vi "Save_Header.vi"() -> ()   [LabVIEW 2018]
uses:
  RxTx/CCS_RxTx.lvclass
  Save Image/Save Image.lvclass
  Channel/Channel.lvclass
panel:
  in  "Stop Button":bool
  out "error out":errorcluster
  in  "Save Image out":refnum<class "Save Image.lvclass">
  in  "RxTx.lvclass":refnum<class "CCS_RxTx.lvclass">
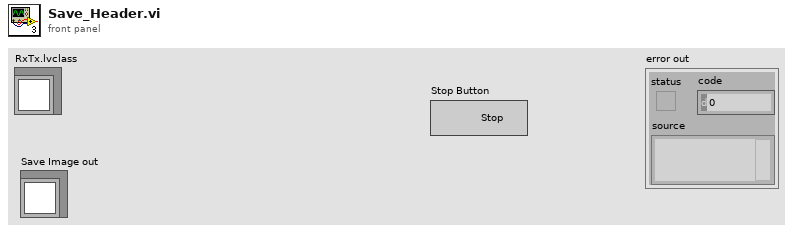
[diagram p1: front panel]
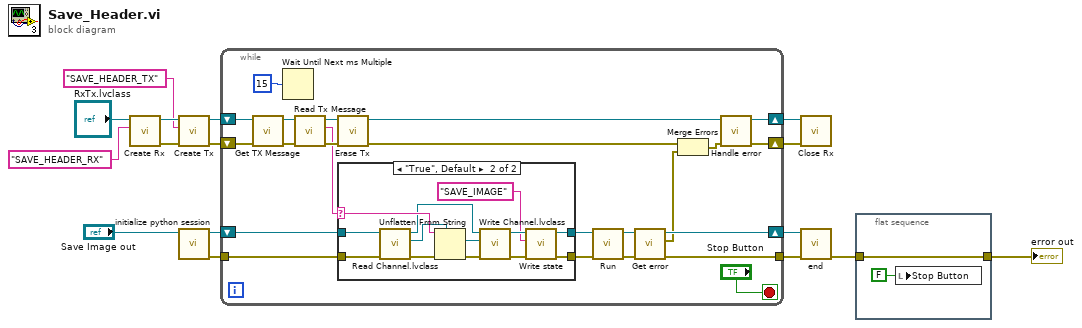
[diagram p0: block diagram]
diagram:
  n1 = call "Create Rx.vi"("Reader Name"="SAVE_HEADER_RX", "RxTx in"="RxTx.lvclass") -> ("error out"=w10:errorcluster, "RxTx out"=w11:refnum<class "CCS_RxTx.lvclass">)  [unwired: 8 in]
  n2 = call "Create Tx.vi"("error in (no error)"=w10, "Writer Name"="SAVE_HEADER_TX" ("Reader Name"), "RxTx in"=w11) -> ("error out"=w3:errorcluster, "RxTx out"=w4:refnum<class "CCS_RxTx.lvclass">)  [unwired: 7 in]
  n3 = call "initialize python session.vi"("Save Image in"="Save Image out") -> ("error out"=w7:errorcluster, "Save Image out"=w14:refnum<class "Save Image.lvclass">)  [unwired: 9 in]
  n4 = while {
    shift-right: [w34] -> w8
    shift-left: w4 -> [w30]
    shift-right: [w19] -> w12
    shift-left: w14 -> [w36]
    shift-right: [w33] -> w5
    shift-left: w3 -> [w29]
    tunnel: w7 -> [w35]
    tunnel: [w20] -> w6
    stop <- "Stop Button" stop-if-true
    n5 = call "Get TX Message.vi"("error in (no error)"=w29, "RxTx in"=w30) -> ("error out"=w28:errorcluster, "RxTx out"=w27:refnum<class "CCS_RxTx.lvclass">)  [unwired: 8 in]
    n6 = Wait Until Next ms Multiple(millisecond multiple=u32 15) -> ()  [unwired: 1 out]
    n7 = call "Read Tx Message.vi"("error in (no error)"=w28, "RxTx in"=w27) -> ("error out"=w25:errorcluster, "Tx Message"=w22:string, "RxTx out"=w26:refnum<class "CCS_RxTx.lvclass">)  [unwired: 7 in]
    n8 = call "Erase Tx.vi"("error in (no error)"=w25, "RxTx in"=w26) -> ("error out"=w24:errorcluster, "RxTx out"=w23:refnum<class "CCS_RxTx.lvclass">)  [unwired: 8 in]
    n9 = case shown="\"True\", Default" w22 {
      selector: w22 -> [_ w54]
      tunnel: [w41 w45] -> w38
      tunnel: [w40 w43] -> w37
      tunnel: w35 -> [w40 w52]
      tunnel: w36 -> [w41 w53]
      frame "", "STOP_APPLICATION" {
      }
      frame "True", Default {
        n10 = call-dynamic "Read Channel.lvclass.vi"("error in (no error)"=w52, "Save Image in"=w53) -> ("error out"=w51:errorcluster, "Channel.lvclass"=w48:refnum<class "Channel.lvclass">, "Save Image out"=w49:refnum<class "Save Image.lvclass">)  [unwired: 7 in]
        n11 = Unflatten From String(type=w48, binary string=w54, error in (no error)=w51) -> (value=w47:refnum<class "Channel.lvclass">, error out=w50:errorcluster)  [unwired: 2 in, 1 out]
        n12 = call-dynamic "Write Channel.lvclass.vi"("error in (no error)"=w50, "Channel.lvclass"=w47, "Save Image in"=w49) -> ("error out"=w44:errorcluster, "Save Image out"=w46:refnum<class "Save Image.lvclass">)  [unwired: 7 in]
        n13 = call "Write state.vi"("error in (no error)"=w44, "String"="SAVE_IMAGE" ("Reader Name"), "Save Image in"=w46) -> ("error out"=w43:errorcluster, "Save Image out"=w45:refnum<class "Save Image.lvclass">)  [unwired: 7 in]
      }
    }
    n14 = call "Run.vi"("error in (no error)"=w37, "Save Image in"=w38) -> ("error out"=w21:errorcluster, "Save Image out"=w18:refnum<class "Save Image.lvclass">)  [unwired: 8 in]
    n15 = call "Get error.vi"("error in (no error)"=w21, "Save Image in"=w18) -> ("error out"=w20:errorcluster, "error"=w17:errorcluster, "Save Image out"=w19:refnum<class "Save Image.lvclass">)  [unwired: 7 in]
    n16 = Merge Errors(w24, w17) -> (w32:errorcluster)
    n17 = call "Handle error.vi"("error in (no error)"=w32, "RxTx in"=w23) -> ("error out"=w33:errorcluster, "RxTx out"=w34:refnum<class "CCS_RxTx.lvclass">)  [unwired: 8 in]
  }
  n18 = call "Close Rx.vi"("error in (no error)"=w5, "RxTx in"=w8) -> ()  [unwired: 8 in, 2 out]
  n19 = call "end.vi"("error in (no error)"=w6, "Save Image in"=w12) -> ("error out"=w2:errorcluster)  [unwired: 8 in, 1 out]
  n20 = flat-sequence {
    tunnel: w2 -> [w56]
    tunnel: [w56] -> w1
    frame #0 {
      n21 = local write "Stop Button"(FALSE ("Stop Button")) -> ()
    }
  }
  "error out" <- w1
